vi "Initialize Tasks.vi"   [LabVIEW 2021, in "Session Management niDAQmx.lvlib"]
uses:
  Session Management niDAQmx.lvlib
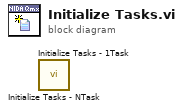
[diagram p0: block diagram]
diagram:
  n1 = call "Initialize Tasks - NTask.vi"() -> ()  [unwired: 8 in, 4 out]
  n2 = call "Initialize Tasks - 1Task.vi"() -> ()  [unwired: 8 in, 4 out]
